vi "FTW-SEQ-Current.vi"(1 "Sequencer":refnum<class "FTW-Sequencer.lvclass">) -> (0 "Current Job":string)   [LabVIEW 2012, in "FTW-Sequencer.lvclass"]
uses:
  FTW-Sequencer.lvclass
  FTW-Sequencer.lvclass/FTW-Sequencer.ctl
panel:
  # "Inputs"
  # "Outputs"
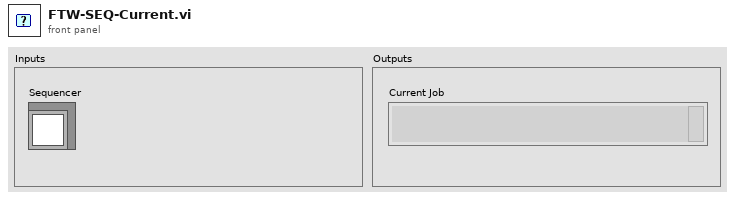
[diagram p1: front panel]
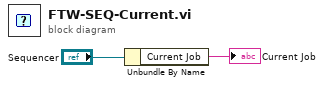
[diagram p0: block diagram]
diagram:
  n1 = Unbundle By Name("Sequencer") -> ("Current Job"=→"Current Job":string)
